vi "niRFUtil MASMT Util All Cosine Window (CDB).vi"(8 "error in (no error)":errorcluster, 9 "scale?":bool, 10 "cosine window":i32(ring) items=["None"=0, "Hanning"=1, "Hamming"=2, "Blackman-Harris"=3, "Exact Blackman"=4, "Blackman"=5, "Flat Top"=6, "4 Term B-Harris"=7, "7 Term B-Harris"=8, "Low Sidelobe"=9, "Blackman Nuttall"=11], 11 "X":cdb[](array[numeric])) -> (0 "error out":errorcluster, 3 "Windowed X":cdb[](array[numeric]))   [LabVIEW 2015, in "niRFUtil.lvlib"]
uses:
  niRFUtil.lvlib
  niRFMASMT_FFT.dll
panel:
  out "WorkH":dbl[](array[numeric])
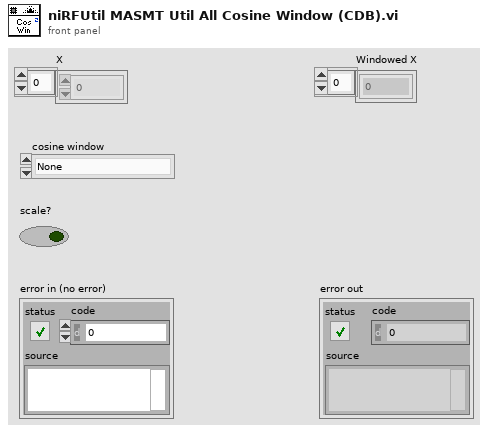
[diagram p1: front panel]
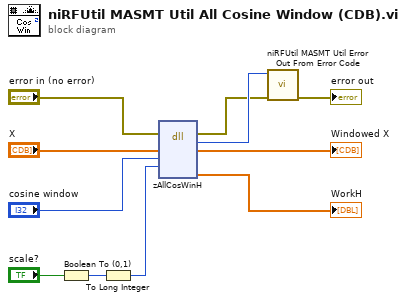
[diagram p0: block diagram]
diagram:
  n1 = Boolean To (0,1)(Boolean="scale?") -> (0, 1=w2:i16)
  n2 = To Long Integer(number=w2) -> (32bit integer=w1:i32)
  n3 = dll-call lib="C:/Perforce/semoore-sales/Customers/NATI-3813/Noise Floor/LV Filters/ParallelComplexFilterRFUtil/niRFUtil/MASMT/Utilities/niRFMASMT_FFT.*" fn="zAllCosWinH"(error in="error in (no error)", "xH"="X", "winType"="cosine window", "scaled"=w1) -> (error out=w6:errorcluster, "return type"=w7:i32, "xH"=→"Windowed X":cdb[], "WorkH"=→"WorkH":dbl[])  [unwired: 5 in, 1 out]
  n4 = call "niRFUtil MASMT Util Error Out From Error Code.vi"("error in (no error)"=w6, "error code"=w7) -> ("error out"=→"error out":errorcluster)  [unwired: 9 in]
